vi "Pack Step Value.vi"(8 "error in (no error)":errorcluster, 10 "Value":string, 11 "O2 Flow Rate STEP in":refnum<class "O2 Flow Rate STEP.lvclass">=refnum) -> (0 "error out":errorcluster, 3 "O2 Flow Rate STEP out":refnum<class "O2 Flow Rate STEP.lvclass">)   [LabVIEW 2014, in "O2 Flow Rate STEP.lvlib" / "O2 Flow Rate STEP.lvclass"]
uses:
  O2 Flow Rate STEP.lvclass
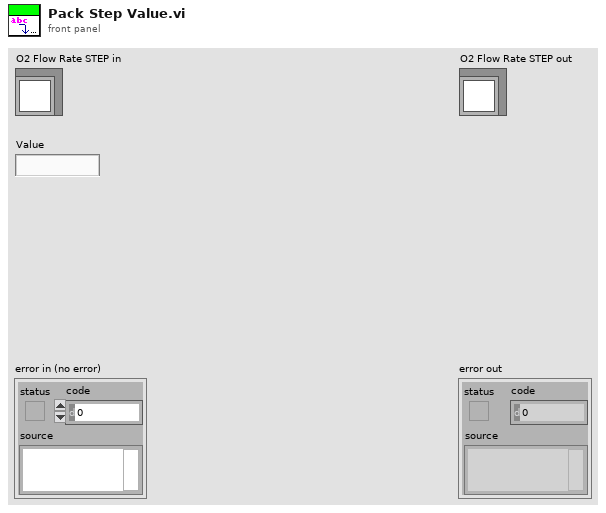
[diagram p1: front panel]
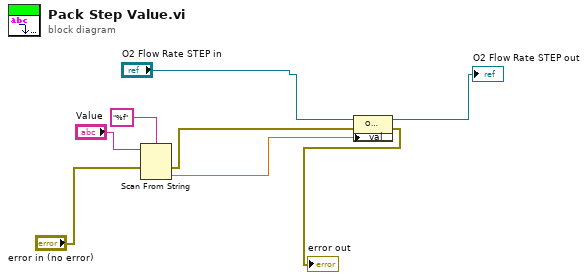
[diagram p0: block diagram]
diagram:
  n1 = Scan From String(format string="%f", input string="Value", error in="error in (no error)") -> (error out=w2:errorcluster, output 1=w3:dbl)  [unwired: 2 in, 2 out]
  n2 = property class="O2 Flow Rate STEP.lvclass"(reference="O2 Flow Rate STEP in", error in=w2, "val"=w3) -> (reference out=→"O2 Flow Rate STEP out":refnum<class "O2 Flow Rate STEP.lvclass">, error out=→"error out":errorcluster)
